vi "Message decoding.vi"(8 "error in (no error)":errorcluster, 10 "Message":string, 11 "TCP Listener in":refnum<class "TCP Listener.lvclass">) -> (0 "error out":errorcluster, 2 "Message decoded":T1, 3 "TCP Listener out":refnum<class "TCP Listener.lvclass">)   [LabVIEW 2026, in "TALOS.lvlib" / "TCP Listener.lvlib" / "TCP Listener.lvclass"]
uses:
  TCP Listener.lvclass
  TCP Writer/TCP Writer/TCP Message Internal Composition.ctl
  TCP Writer/TCP Writer/TCP Message.ctl
  TCP Writer/TCP Writer/TCP Writer.lvclass
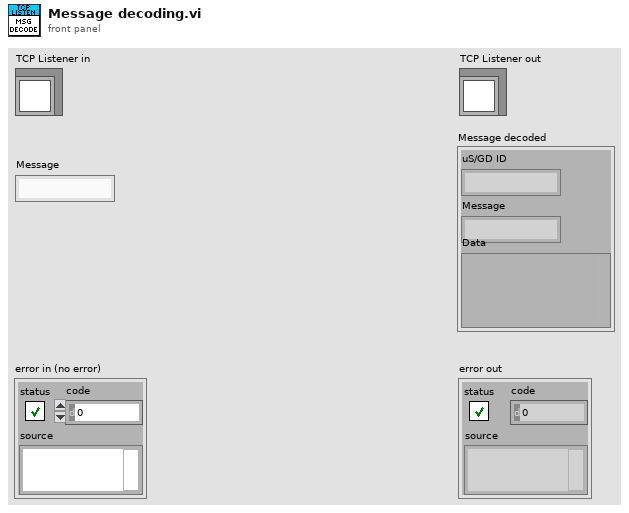
[diagram p1: front panel]
types:
  T1 = typedef "TALOS.lvlib/TCP Writer.lvlib/TCP Writer.lvclass/TCP Message Internal Composition.ctl" = cluster{"uS/GD ID":string, "Message":string, "Data":variant}
  T2 = typedef "TALOS.lvlib/TCP Writer.lvlib/TCP Writer.lvclass/TCP Message.ctl" = cluster{"Type string":i16[], "Data string":string}
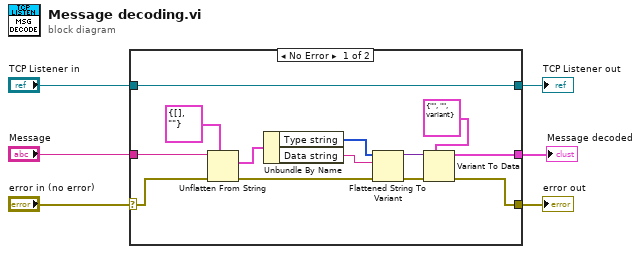
[diagram p0: block diagram]
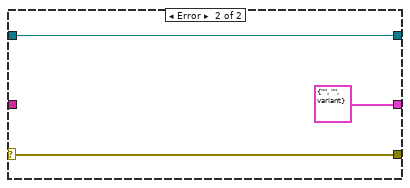
[diagram p2: hidden frame]
diagram:
  n1 = case shown="No Error" "error in (no error)" {
    selector: "error in (no error)" -> [w18 w22]
    tunnel: [w16 w22] -> w5
    tunnel: [w19 w21] -> w3
    tunnel: "TCP Listener in" -> [w19 w21]
    tunnel: "Message" -> [w15 _]
    tunnel: [w17 T1 {"uS/GD ID"="", "Message"="", "Data"=variant}] -> w1
    frame No Error {
      n2 = Unflatten From String(type=T2 {"Type string"=[], "Data string"=""}, binary string=w15, error in (no error)=w18) -> (value=w12:T2, error out=w13:errorcluster)  [unwired: 2 in, 1 out]
      n3 = Unbundle By Name(w12) -> ("Type string"=w7:i16[], "Data string"=w8:string)
      n4 = Flattened String To Variant(4:w13, 6:w8, 7:w7) -> (0:w11:errorcluster, 3:w9:variant)
      n5 = Variant To Data(error in=w11, type=T1 {"uS/GD ID"="", "Message"="", "Data"=variant}, Variant=w9) -> (data=w17:T1, error out=w16:errorcluster)
    }
    frame Error {
    }
  }
  "error out" <- w5
  "TCP Listener out" <- w3
  "Message decoded" <- w1
